vi "exersise 3-6.vi"() -> ()   [LabVIEW 2014]
panel:
  in  "stop":bool
  in  "Ring":u16(ring) items=["Fahrenheit to Celsius", " Celsius to Kelvin", "Fahrenheit to Kelvin", "Celsius to Fahrenheit"]
  out "value unknown":dbl
  in  "value known":dbl
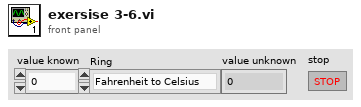
[diagram p1: front panel]
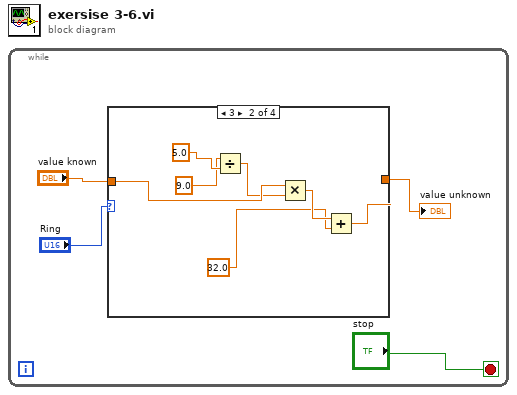
[diagram p0: block diagram]
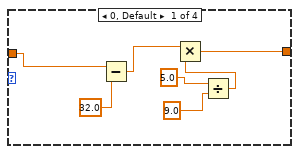
[diagram p2: hidden frame]
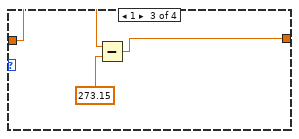
[diagram p3: hidden frame]
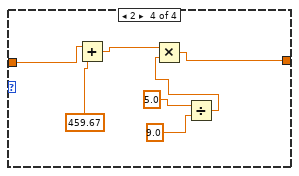
[diagram p4: hidden frame]
diagram:
  n1 = while {
    stop <- "stop" stop-if-true
    n2 = case shown="3" "Ring" {
      tunnel: "value known" -> [w6 w18 w20 w26]
      tunnel: [w5 w14 w19 w22] -> w2
      frame 0, Default {
        n3 = Subtract(x=w6, y=32.0) -> (x-y=w9:dbl)
        n4 = Divide(x=5.0, y=9.0) -> (x/y=w8:dbl)
        n5 = Multiply(x=w9, y=w8) -> (x*y=w5:dbl)
      }
      frame 3 {
        n6 = Divide(x=9.0, y=5.0) -> (x/y=w17:dbl)
        n7 = Multiply(x=w18, y=w17) -> (x*y=w16:dbl)
        n8 = Add(x=w16, y=32.0) -> (x+y=w14:dbl)
      }
      frame 1 {
        n9 = Subtract(x=w20, y=273.15) -> (x-y=w19:dbl)
      }
      frame 2 {
        n10 = Add(x=w26, y=459.67) -> (x+y=w23:dbl)
        n11 = Divide(x=5.0, y=9.0) -> (x/y=w24:dbl)
        n12 = Multiply(x=w23, y=w24) -> (x*y=w22:dbl)
      }
    }
    "value unknown" <- w2
  }
